vi "GlobalArduino.vi"() -> ()   [LabVIEW 2012]
panel:
  out "semaphore read":T1
  out "semaphore":T1
  in  "Last position command time":u64[](array[numeric])
  out "VISA resource name out":refnum<visa-resource-name>
  out "error out":errorcluster
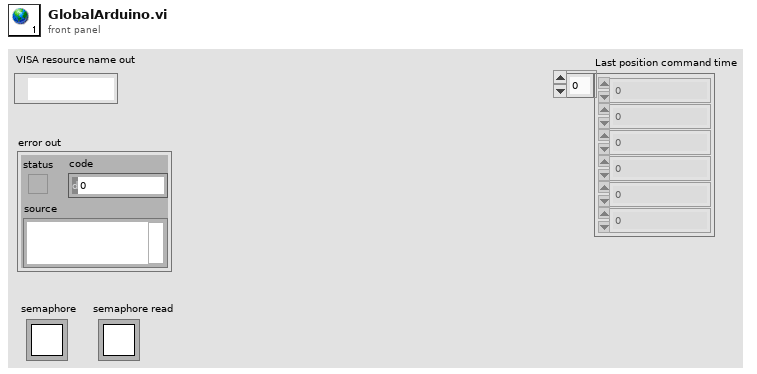
[diagram p1: front panel]
types:
  T1 = typedef "Semaphore RefNum" = refnum<k1>
diagram:
